vi "2DGenerator.vi"(8 "Do That":bool, 10 "Colum":i32, 11 "Row":i32) -> (3 "2D Array":u64[][](array[numeric]))   [LabVIEW 2023]
uses:
  <vilib>/numeric/Random Number (Range) U64.vi
  <vilib>/numeric/sub_Random U32.vi
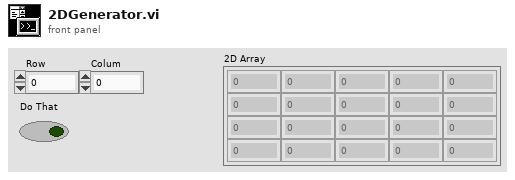
[diagram p1: front panel]
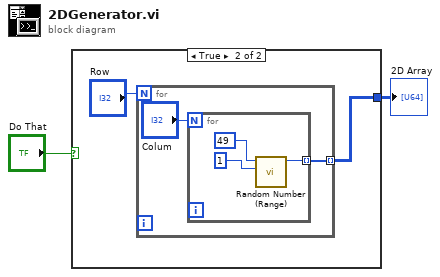
[diagram p0: block diagram]
diagram:
  n1 = case shown="True" "Do That" {
    tunnel: [_ w4] -> w1
    frame False {
    }
    frame True {
      n2 = for {
        N: "Row" -> [_]
        tunnel: [w6] -> w4 mode=indexing
        n3 = for {
          N: "Colum" -> [_]
          tunnel: [w7] -> w6 mode=indexing
          n4 = call-poly <vilib>:"Random Number (Range).vi"("lower bound (0)"=u64 1, "upper bound (100)"=u64 49) -> ("number"=w7:u64)  [unwired: 9 in]
        }
      }
    }
  }
  "2D Array" <- w1
